vi "Append to filename base.vi"(3 "Text to append to base":string="_APPENDED TEXT", 4 "Path":path=path "C:/myfiles.are.here.Text") -> (1 "Path out":path=path "C:/myfiles.are.here_APPENDED TEXT.Text")   [LabVIEW 2013]
doc: "This .vi adds text to the filename base, right before the \".\" and the extension."
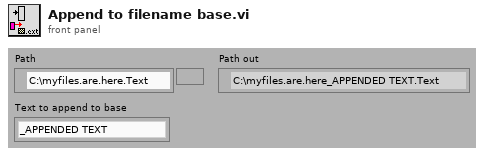
[diagram p1: front panel]
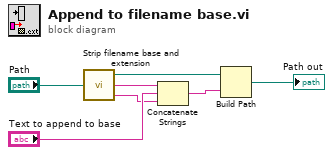
[diagram p0: block diagram]
diagram:
  n1 = call "Strip filename base and extension.vi"("Path"="Path") -> ("stripped path"=w2:path, "Filename base"=w6:string, "Filename extension (.txt)"=w4:string)
  n2 = Concatenate Strings(w6, "Text to append to base", w4) -> (w3:string)
  n3 = Build Path(base path=w2, name or relative path=w3) -> (appended path=→"Path out":path)
